vi "auto_v1.vi"() -> ()   [LabVIEW 2012]
uses:
  SubVIs/auto_drive_TYP.ctl
  SubVIs/State_Typ.ctl
  <vilib>/NXT/Hardware/Plugins/Tetrix DC Motor/TetrixDCMotorAddress.ctl
  <vilib>/NXT/Dual Mode Library/Waits/Wait_Num(msec).vi
  <vilib>/NXT/NXTIO Xnodes/NXTIONodeSubVIs/TETRIX IO Check Battery.vi
  <vilib>/NXT/Dual Mode Library/Display/drawNumber.vi
  <vilib>/NXT/NXTIO Xnodes/NXTIONodeSubVIs/TETRIX IO Stop DC Motors.vi
  <vilib>/NXT/Dual Mode Library/Sound/Tone.vi
  <vilib>/NXT/Dual Mode Library/Waits/Wait_Num.vi
  <vilib>/NXT/Subs/LVHSConnector.ctl
  <vilib>/NXT/NXTIO Xnodes/AddressXNode/NXTIOAddress.xnode
  <vilib>/NXT/NXTIO Xnodes/NXTIOXNode/NXTIO.xnode
  Mecanum Drive.lvrbt
  <vilib>/NXT/LegoClasses/BrickReference/BrickReference.lvclass
panel:
  out "Enabled":bool
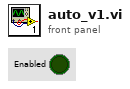
[diagram p1: front panel]
types:
  T1 = typedef "auto_drive_TYP.ctl" = cluster{"Left X":i8, "Left Y":i8, "Right X":i8, "Power (100)":i8, "Wait (ms)":u32}
  T2 = typedef "State_Typ.ctl" = enum16{"Move", "Check for Position 2", "Check for Position 3", "Stop"}
  T3 = typedef "TetrixDCMotorAddress.ctl" = i32
  T4 = typedef "LVHSConnector.ctl" = refnum<class "BrickReference.lvclass">
  T5 = cluster{"TetrixDCMotor":T3, "TetrixDCMotor 2":T3}
  T6 = cluster{"Direction (0-9)":i16, "Signal Strength (Array)":u8[]}
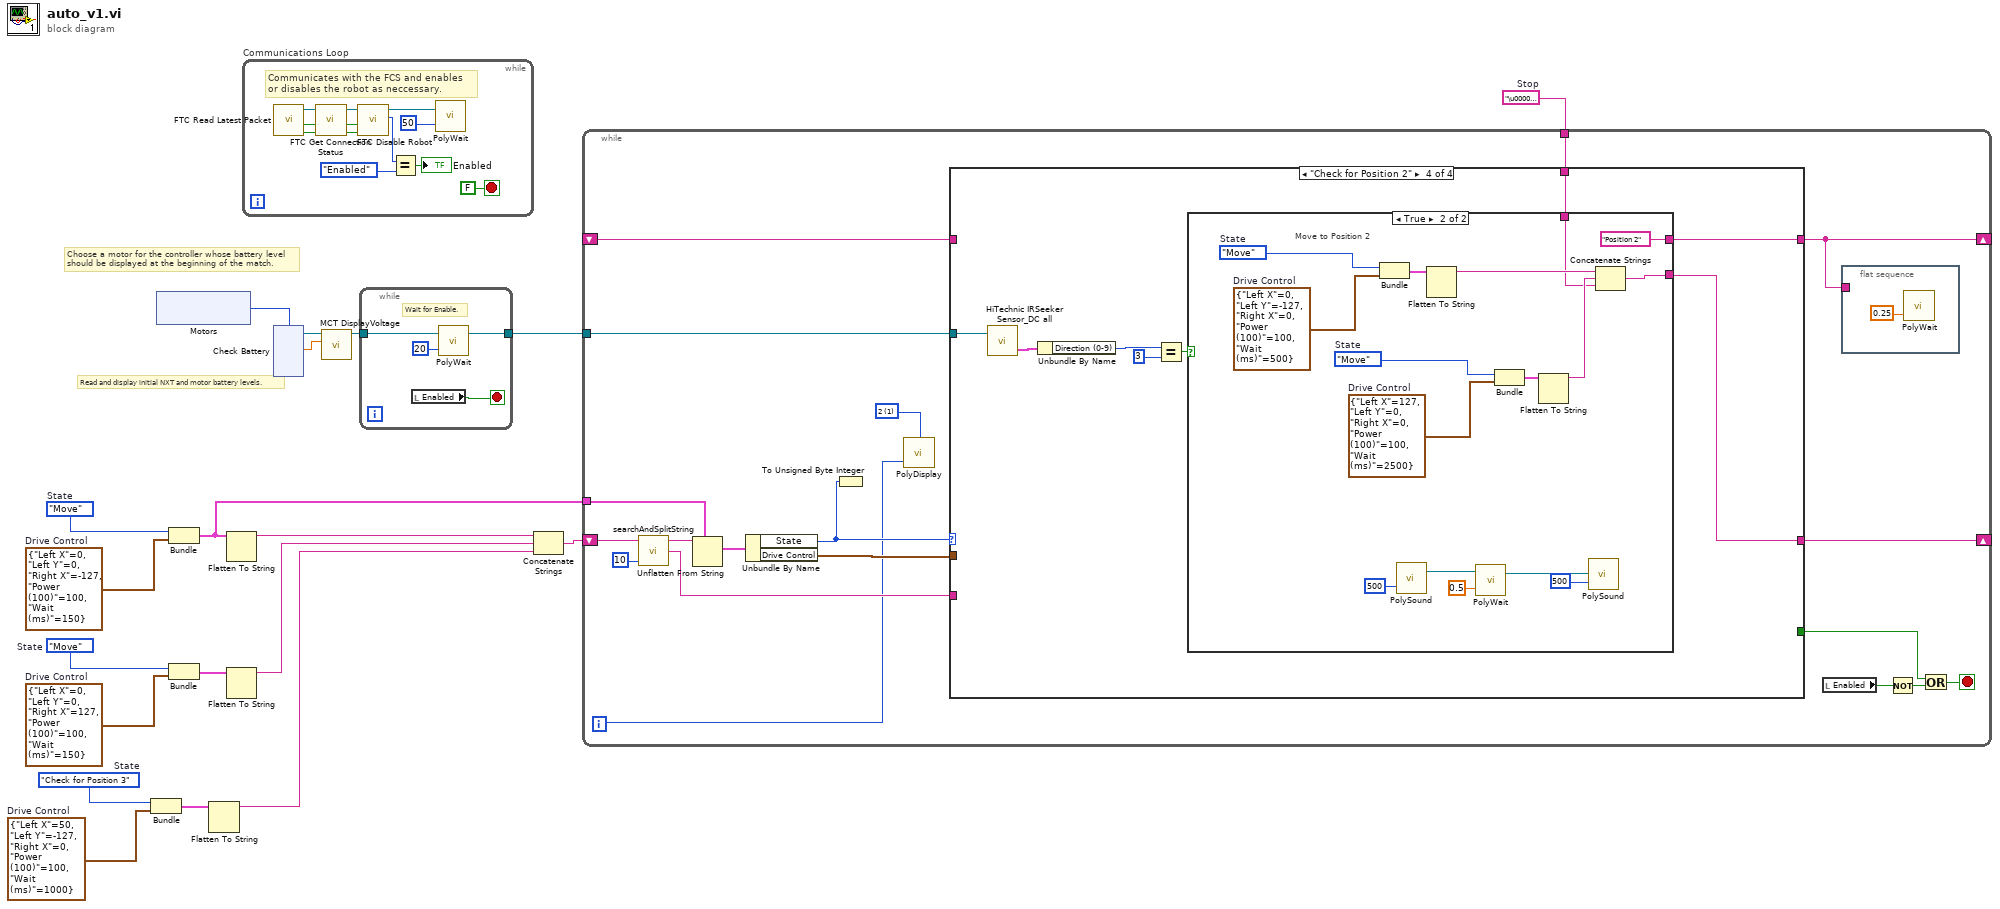
[diagram p0: block diagram]
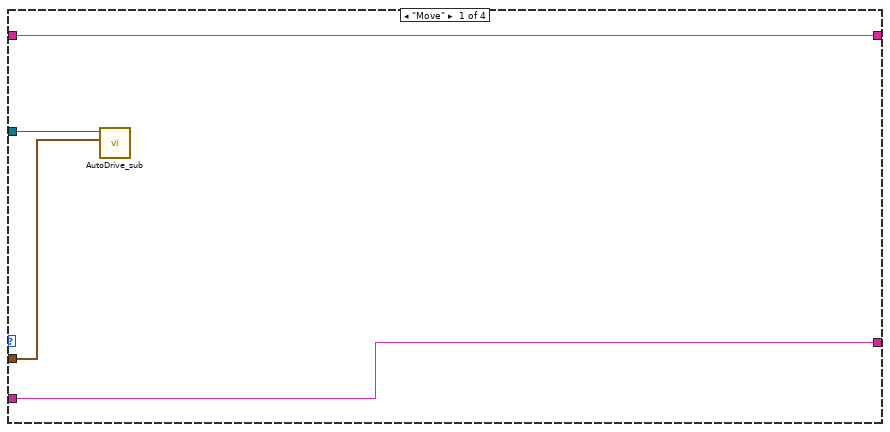
[diagram p2: hidden frame]
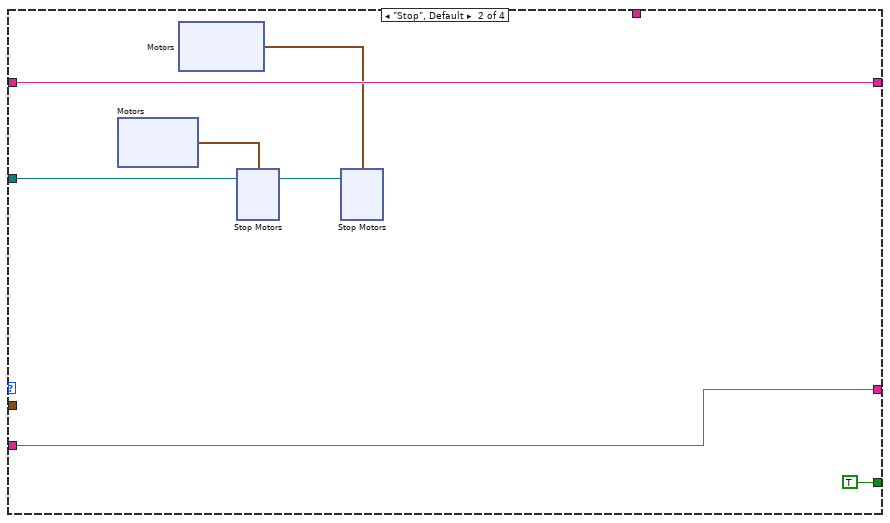
[diagram p3: hidden frame]
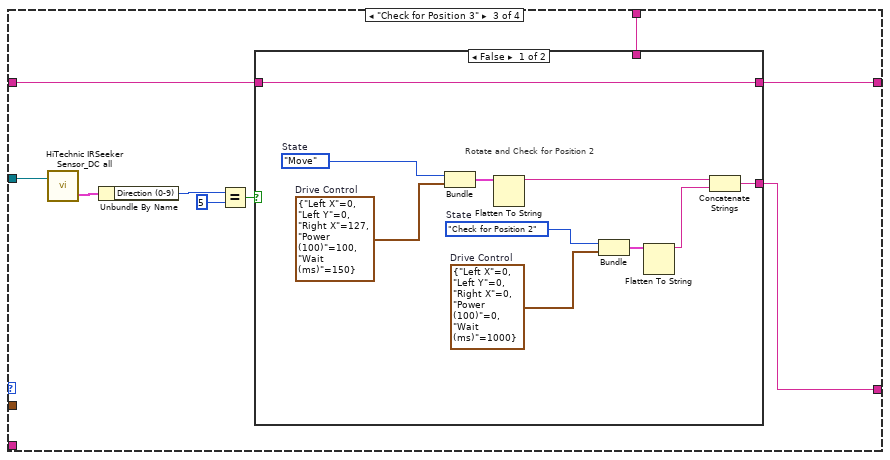
[diagram p4: hidden frame]
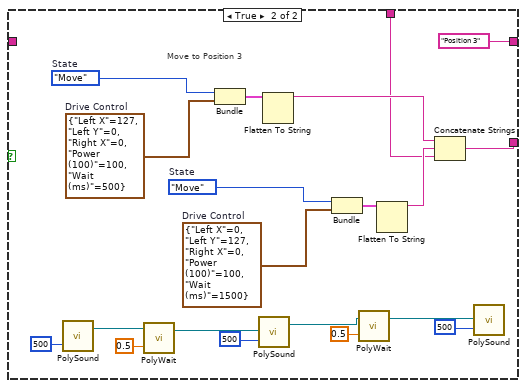
[diagram p5: hidden frame]
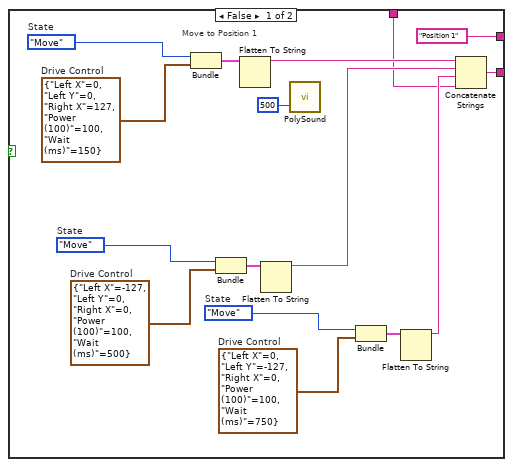
[diagram p6: hidden frame]
diagram:
  w6 = T1 {"Left X"=0, "Left Y"=0, "Right X"=127, "Power (100)"=100, "Wait (ms)"=150}  # Drive Control
  w5 = State_Typ."Move"  # State
  w9 = T1 {"Left X"=0, "Left Y"=0, "Right X"=-127, "Power (100)"=100, "Wait (ms)"=150}  # Drive Control
  w10 = State_Typ."Move"  # State
  w15 = "\u0000\u0003\u0000\u0000d\u0000\u0000\u0000–"  # Stop
  w16 = State_Typ."Check for Position 3"  # State
  w18 = T1 {"Left X"=50, "Left Y"=-127, "Right X"=0, "Power (100)"=100, "Wait (ms)"=1000}  # Drive Control
  # "Read and display initial NXT and motor battery levels."
  # "Choose a motor for the controller whose battery level \nshould be displayed at the beginning of the match."
  n1 = Bundle("State"=w16, "Drive Control"=w18) -> (w17:cluster{"State":T2, "Drive Control":T1})  [unwired: 1 in]
  n2 = xnode "Motors"() -> ("Motor"=w11:T3)
  n3 = Bundle("State"=w10, "Drive Control"=w9) -> (w8:cluster{"State":T2, "Drive Control":T1})  [unwired: 1 in]
  n4 = Bundle("State"=w5, "Drive Control"=w6) -> (w7:cluster{"State":T2, "Drive Control":T1})  [unwired: 1 in]
  n5 = Flatten To String(anything=w17) -> (data string=w2:string)  [unwired: 3 in, 2 out]
  n6 = Flatten To String(anything=w8) -> (data string=w3:string)  [unwired: 3 in, 2 out]
  n7 = Flatten To String(anything=w7) -> (data string=w4:string)  [unwired: 3 in, 2 out]
  n8 = while "Communications Loop" {
    stop <- FALSE stop-if-true
    # "Communicates with the FCS and enables \nor disables the robot as neccessary."
    n9 = call <vilib>:"FTC Read Latest Packet.vi"() -> ("Packet Received?"=w29:bool, "Stopped?"=w28:bool, "NXT/EV3"=w31:T4)  [unwired: 6 in, 3 out]
    n10 = call <vilib>:"FTC Get Connection Status.vi"("Packet Received?"=w29, "Stopped?"=w28, "NXT/EV3"=w31) -> ("Online?"=w20:bool, "Stopped?"=w21:bool, "NXT/EV3"=w30:T4)  [unwired: 5 in]
    n11 = call <vilib>:"FTC Disable Robot.vi"("Online?"=w20, "Stopped?"=w21, "NXT/EV3"=w30) -> ("Enabled?"=w24:enum16{"Disabled", "Enabled"}, "NXT/EV3"=w26:T4)  [unwired: 3 in]
    n12 = Equal?(x=w24, y=enum16{"Disabled", "Enabled"}."Enabled") -> (x = y?=→"Enabled":bool)
    n13 = call-poly <vilib>:"PolyWait.vi"("Time (100 msec)"=u32 50 ("Time (msec)"), "NXT/EV3"=w26) -> ()  [unwired: 2 in, 1 out]
  }
  n14 = xnode "Check Battery"("Motors"=w11) -> ("Voltage 1"=w12:sgl, "NXT/EV3"=w14:T4)  [unwired: 1 in]
  n15 = call <vilib>:"MCT DisplayVoltage.vi"("Motor Voltage"=w12, "NXT/EV3"=w14) -> ("NXT/EV3"=w13:T4)  [unwired: 9 in]
  n16 = while {
    tunnel: [w33] -> w19
    tunnel: w13 -> [w32]
    stop <- w34 stop-if-true
    # "Wait for Enable."
    n17 = local read "Enabled"() -> (w34:bool)
    n18 = call-poly <vilib>:"PolyWait.vi"("Time (100 msec)"=u32 20 ("Time (msec)"), "NXT/EV3"=w32) -> ("NXT/EV3"=w33:T4)  [unwired: 2 in]
  }
  n19 = Concatenate Strings(w3, w4, w2) -> (w1:string)
  n20 = while {
    tunnel: w19 -> [w54]
    shift-right: [w45] -> _
    shift-left: w1 -> [w43]
    tunnel: w8 -> [w46]
    shift-right: [w36] -> _
    shift-left: _ -> [w44]
    tunnel: w15 -> [w41]
    i -> [w37]
    stop <- w53 stop-if-true
    w38 = i16 1 items=["1", "2", "3", "4", "5", "6", "7", "8", "9", "10", "11", "12"] ("Line")
    n21 = call <vilib>:"searchAndSplitString.vi"("offset (0)"=10 ("length (rest)"), "string"=w43) -> ("match + rest of string"=w42:string, "substring before match"=w48:string)  [unwired: 1 in, 1 out]
    n22 = Unflatten From String(type=w46, binary string=w48) -> (value=w47:cluster{"State":T2, "Drive Control":T1})  [unwired: 3 in, 2 out]
    n23 = Unbundle By Name(w47) -> ("State"=w39:T2, "Drive Control"=w49:T1)
    n24 = To Unsigned Byte Integer(number=w39) -> ()  [unwired: 1 out]
    n25 = call-poly <vilib>:"PolyDisplay.vi"("number"=w37, "Line"=w38) -> ()  [unwired: 2 in, 1 out]
    n26 = case shown="\"Check for Position 2\"" w39 {
      tunnel: w54 -> [w59 w66 w84 w122]
      tunnel: [_ TRUE _ _] -> w52
      tunnel: w49 -> [w58 _ _ _]
      tunnel: w42 -> [w57 w64 _ _]
      tunnel: [w57 w64 w79 w118] -> w45
      tunnel: [w56 w63 w82 w120] -> w36
      tunnel: w44 -> [w56 w63 w81 _]
      tunnel: w41 -> [_ _ w80 w119]
      frame "Move" {
        n27 = call "AutoDrive_sub.vi"("Drive Control"=w58, "NXT/EV3"=w59) -> ()  [unwired: 9 in, 1 out]
      }
      frame "Stop", Default {
        n28 = xnode "Motors"() -> ("Motor"=w62:cluster{"TetrixDCMotor":T3, "TetrixDCMotor":T3})
        n29 = xnode "Motors"() -> ("Motor"=w61:cluster{"TetrixDCMotor":T3, "TetrixDCMotor":T3})
        n30 = xnode "Stop Motors"("Motors"=w62, "NXT/EV3"=w66) -> ("NXT/EV3"=w60:T4)
        n31 = xnode "Stop Motors"("Motors"=w61, "NXT/EV3"=w60) -> ()  [unwired: 1 out]
      }
      frame "Check for Position 3" {
        n32 = call <vilib>:"HiTechnic IRSeeker Sensor_DC all.vi"("NXT/EV3"=w84) -> ("All Info"=w87:T6)  [unwired: 2 in, 1 out]
        n33 = Unbundle By Name(w87) -> ("Direction (0-9)"=w85:i16)
        n34 = Equal?(x=w85, y=i16 5) -> (x = y?=w83:bool)
        n35 = case shown="False" w83 {
          tunnel: [w89 w109] -> w79
          tunnel: [w88 "Position 3"] -> w82
          tunnel: w81 -> [w88 _]
          tunnel: w80 -> [_ w107]
          frame False {
            w94 = T1 {"Left X"=0, "Left Y"=0, "Right X"=0, "Power (100)"=0, "Wait (ms)"=1000}  # Drive Control
            w95 = State_Typ."Check for Position 2"  # State
            w91 = T1 {"Left X"=0, "Left Y"=0, "Right X"=127, "Power (100)"=100, "Wait (ms)"=150}  # Drive Control
            w90 = State_Typ."Move"  # State
            # "Rotate and Check for Position 2"
            n36 = Bundle("State"=w90, "Drive Control"=w91) -> (w92:cluster{"State":T2, "Drive Control":T1})  [unwired: 1 in]
            n37 = Flatten To String(anything=w92) -> (data string=w97:string)  [unwired: 3 in, 2 out]
            n38 = Bundle("State"=w95, "Drive Control"=w94) -> (w93:cluster{"State":T2, "Drive Control":T1})  [unwired: 1 in]
            n39 = Flatten To String(anything=w93) -> (data string=w96:string)  [unwired: 3 in, 2 out]
            n40 = Concatenate Strings(w97, w96) -> (w89:string)
          }
          frame True {
            w114 = T1 {"Left X"=0, "Left Y"=127, "Right X"=0, "Power (100)"=100, "Wait (ms)"=1500}  # Drive Control
            w115 = State_Typ."Move"  # State
            w117 = T1 {"Left X"=127, "Left Y"=0, "Right X"=0, "Power (100)"=100, "Wait (ms)"=500}  # Drive Control
            w116 = State_Typ."Move"  # State
            # "Move to Position 3"
            n41 = call-poly <vilib>:"PolySound.vi"("Duration (500 ms)"=u16 500) -> ("NXT/EV3"=w103:T4)  [unwired: 3 in]
            n42 = call-poly <vilib>:"PolyWait.vi"("Time (1 sec)"=sgl 0.5, "NXT/EV3"=w103) -> ("NXT/EV3"=w102:T4)  [unwired: 2 in]
            n43 = Bundle("State"=w116, "Drive Control"=w117) -> (w113:cluster{"State":T2, "Drive Control":T1})  [unwired: 1 in]
            n44 = call-poly <vilib>:"PolySound.vi"("Duration (500 ms)"=u16 500, "NXT/EV3"=w102) -> ("NXT/EV3"=w99:T4)  [unwired: 2 in]
            n45 = Flatten To String(anything=w113) -> (data string=w110:string)  [unwired: 3 in, 2 out]
            n46 = Bundle("State"=w115, "Drive Control"=w114) -> (w112:cluster{"State":T2, "Drive Control":T1})  [unwired: 1 in]
            n47 = call-poly <vilib>:"PolyWait.vi"("Time (1 sec)"=sgl 0.5, "NXT/EV3"=w99) -> ("NXT/EV3"=w98:T4)  [unwired: 2 in]
            n48 = Flatten To String(anything=w112) -> (data string=w111:string)  [unwired: 3 in, 2 out]
            n49 = Concatenate Strings(w110, w111, w107) -> (w109:string)
            n50 = call-poly <vilib>:"PolySound.vi"("Duration (500 ms)"=u16 500, "NXT/EV3"=w98) -> ()  [unwired: 2 in, 1 out]
          }
        }
      }
      frame "Check for Position 2" {
        n51 = call <vilib>:"HiTechnic IRSeeker Sensor_DC all.vi"("NXT/EV3"=w122) -> ("All Info"=w125:T6)  [unwired: 2 in, 1 out]
        n52 = Unbundle By Name(w125) -> ("Direction (0-9)"=w123:i16)
        n53 = Equal?(x=w123, y=i16 3) -> (x = y?=w121:bool)
        n54 = case shown="True" w121 {
          tunnel: [w138 w149] -> w118
          tunnel: ["Position 1" "Position 2"] -> w120
          tunnel: w119 -> [w126 w142]
          frame False {
            w133 = T1 {"Left X"=-127, "Left Y"=0, "Right X"=0, "Power (100)"=100, "Wait (ms)"=500}  # Drive Control
            w134 = State_Typ."Move"  # State
            w136 = T1 {"Left X"=0, "Left Y"=-127, "Right X"=0, "Power (100)"=100, "Wait (ms)"=750}  # Drive Control
            w137 = State_Typ."Move"  # State
            w140 = T1 {"Left X"=0, "Left Y"=0, "Right X"=127, "Power (100)"=100, "Wait (ms)"=150}  # Drive Control
            w141 = State_Typ."Move"  # State
            # "Move to Position 1"
            n55 = Bundle("State"=w141, "Drive Control"=w140) -> (w139:cluster{"State":T2, "Drive Control":T1})  [unwired: 1 in]
            n56 = Bundle("State"=w134, "Drive Control"=w133) -> (w132:cluster{"State":T2, "Drive Control":T1})  [unwired: 1 in]
            n57 = Flatten To String(anything=w139) -> (data string=w128:string)  [unwired: 3 in, 2 out]
            n58 = Flatten To String(anything=w132) -> (data string=w131:string)  [unwired: 3 in, 2 out]
            n59 = call-poly <vilib>:"PolySound.vi"("Duration (500 ms)"=u16 500) -> ()  [unwired: 3 in, 1 out]
            n60 = Bundle("State"=w137, "Drive Control"=w136) -> (w135:cluster{"State":T2, "Drive Control":T1})  [unwired: 1 in]
            n61 = Flatten To String(anything=w135) -> (data string=w130:string)  [unwired: 3 in, 2 out]
            n62 = Concatenate Strings(w128, w131, w130, w126) -> (w138:string)
          }
          frame True {
            w153 = T1 {"Left X"=127, "Left Y"=0, "Right X"=0, "Power (100)"=100, "Wait (ms)"=2500}  # Drive Control
            w152 = State_Typ."Move"  # State
            w150 = T1 {"Left X"=0, "Left Y"=-127, "Right X"=0, "Power (100)"=100, "Wait (ms)"=500}  # Drive Control
            w151 = State_Typ."Move"  # State
            # "Move to Position 2"
            n63 = Bundle("State"=w151, "Drive Control"=w150) -> (w154:cluster{"State":T2, "Drive Control":T1})  [unwired: 1 in]
            n64 = call-poly <vilib>:"PolySound.vi"("Duration (500 ms)"=u16 500) -> ("NXT/EV3"=w144:T4)  [unwired: 3 in]
            n65 = Flatten To String(anything=w154) -> (data string=w157:string)  [unwired: 3 in, 2 out]
            n66 = call-poly <vilib>:"PolyWait.vi"("Time (1 sec)"=sgl 0.5, "NXT/EV3"=w144) -> ("NXT/EV3"=w143:T4)  [unwired: 2 in]
            n67 = Bundle("State"=w152, "Drive Control"=w153) -> (w155:cluster{"State":T2, "Drive Control":T1})  [unwired: 1 in]
            n68 = Flatten To String(anything=w155) -> (data string=w156:string)  [unwired: 3 in, 2 out]
            n69 = call-poly <vilib>:"PolySound.vi"("Duration (500 ms)"=u16 500, "NXT/EV3"=w143) -> ()  [unwired: 2 in, 1 out]
            n70 = Concatenate Strings(w157, w156, w142) -> (w149:string)
          }
        }
      }
    }
    n71 = local read "Enabled"() -> (w51:bool)
    n72 = flat-sequence {
      tunnel: w36 -> [_]
      frame #0 {
        n73 = call-poly <vilib>:"PolyWait.vi"("Time (1 sec)"=sgl 0.25) -> ()  [unwired: 3 in, 1 out]
      }
    }
    n74 = Not(x=w51) -> (.not. x?=w40:bool)
    n75 = Or(x=w52, y=w40) -> (x .or. y?=w53:bool)
  }
